vi "Actor Core.vi"(8 "error in":errorcluster, 11 "AverageCollector2D in":refnum<class "AverageCollector2D.lvclass">) -> (0 "error out":errorcluster, 3 "Actor out":refnum<class "Actor.lvclass">)   [LabVIEW 2014, in "AverageCollector2D.lvclass"]
doc: "(<B>Filename</B>: Actor Framework.lvlib:Actor.lvclass:Actor Core.vi)\n\nReceives messages to the actor, reacts to them, and initiates any error handling that may shut the actor down.\n\nDescendant classes may override this VI to append parallel tasks for the actor to complete while it handles messages. Overrides use the Call Parent Method node."
uses:
  AverageCollector2D.lvclass
  Framework/Collector/AbstractCollector2D/AbstractCollector2D.lvclass
  Framework/Interfaces/Viewable Actor/Viewable Actor.lvclass
  <vilib>/ActorFramework/Message Enqueuer/Message Priority.ctl
  <vilib>/ActorFramework/Message Enqueuer/Message Enqueuer.lvclass
  Framework/Collector/AbstractCollector/AbstractCollector Messages/Write Needed Number Msg/Write Needed Number Msg.lvclass
  Framework/Collector/AbstractCollector/AbstractCollector Messages/Reset Msg/Reset Msg.lvclass
  <vilib>/ActorFramework/Actor/Actor.lvclass
  Framework/Interfaces/Observable Actor/Observable Actor.lvclass
  Framework/Collector/AbstractCollector/AbstractCollector.lvclass
  Framework/Model/Data/Data2D/Data2D.lvclass
  Framework/Collector/AbstractCollector2D/Data2D Cluster.ctl
panel:
  out "Collected number":u32
  out "Stop":bool=TRUE
  in  "Needed number":u32=1
  in  "Reset":bool
  out "Intermediate result":dbl[][](graph)
  out "Data in":dbl[][](graph)
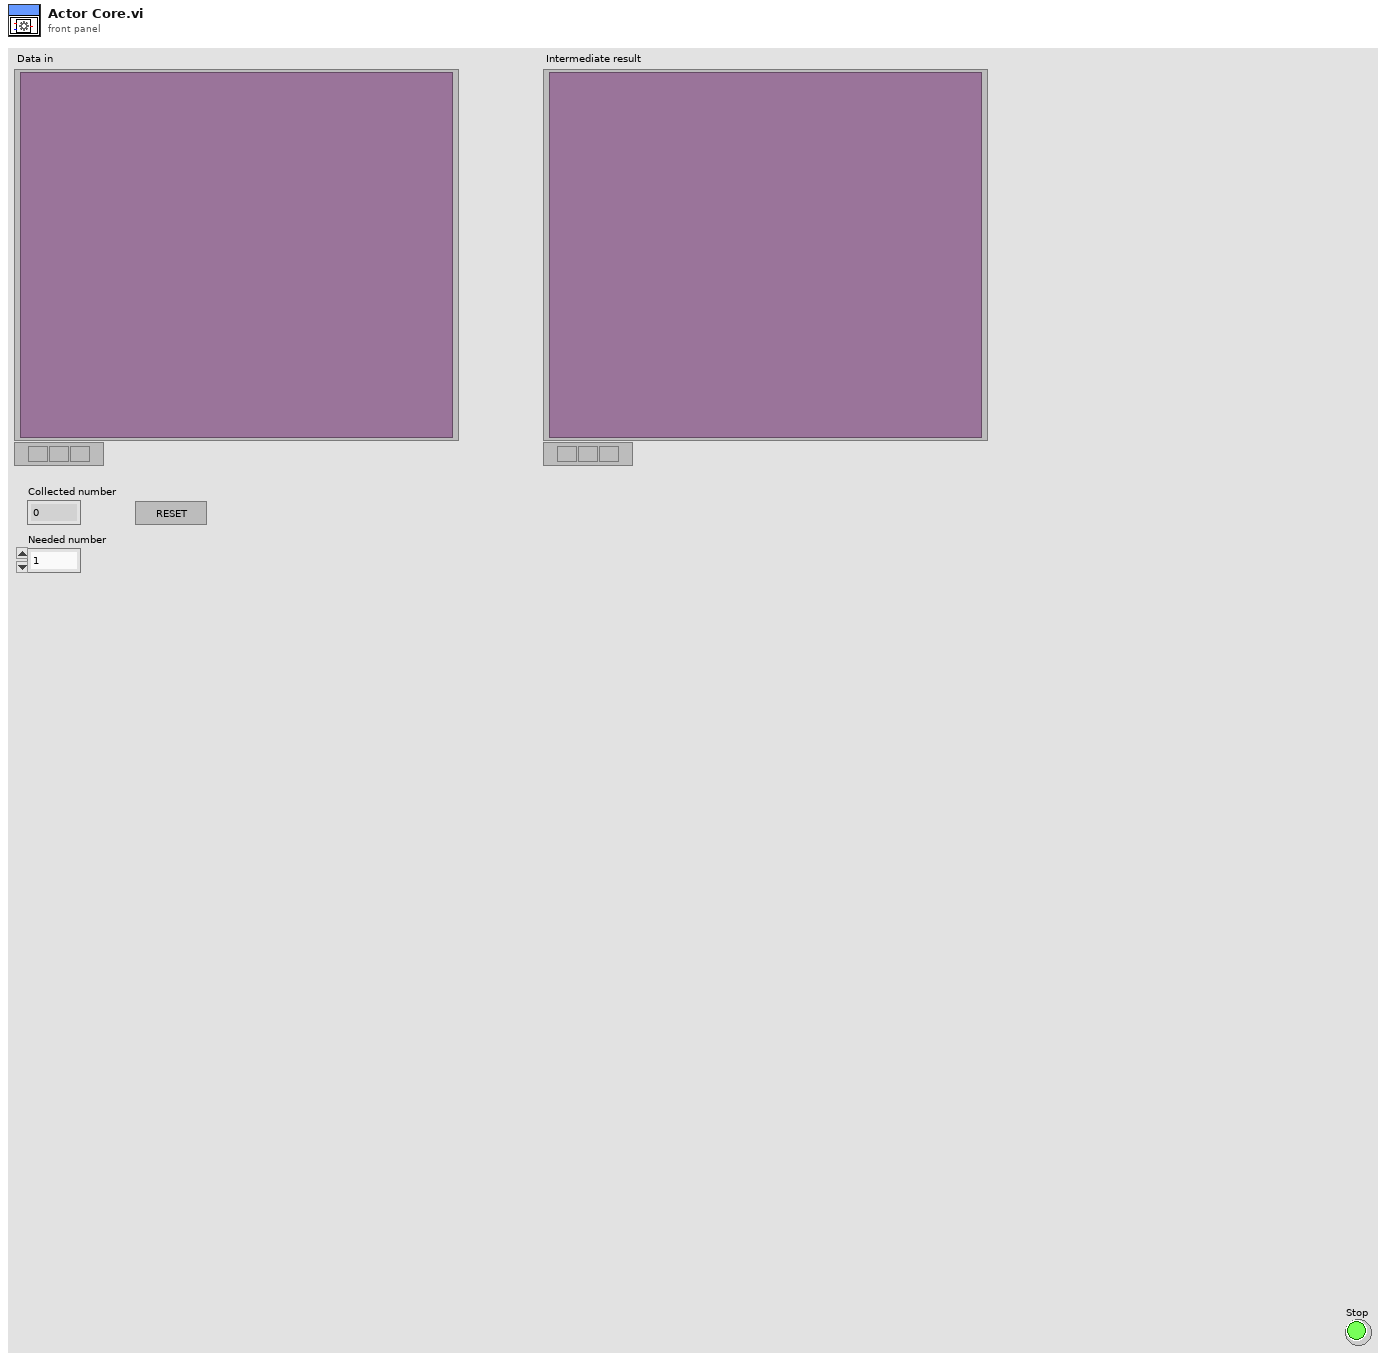
[diagram p1: front panel]
types:
  T1 = typedef "Observable Actor.lvlib/Observable Actor.lvclass/Observer.ctl" = refnum<queue>
  T2 = typedef "AbstractCollector2D.lvclass/Data2D Cluster.ctl" = cluster{"in":refnum<class "Data2D.lvclass">, "intermediate":refnum<class "Data2D.lvclass">}
  T3 = typedef "Actor Framework.lvlib/Message Enqueuer.lvclass/Message Priority.ctl" = enum16{"Low", "Normal", "High"}
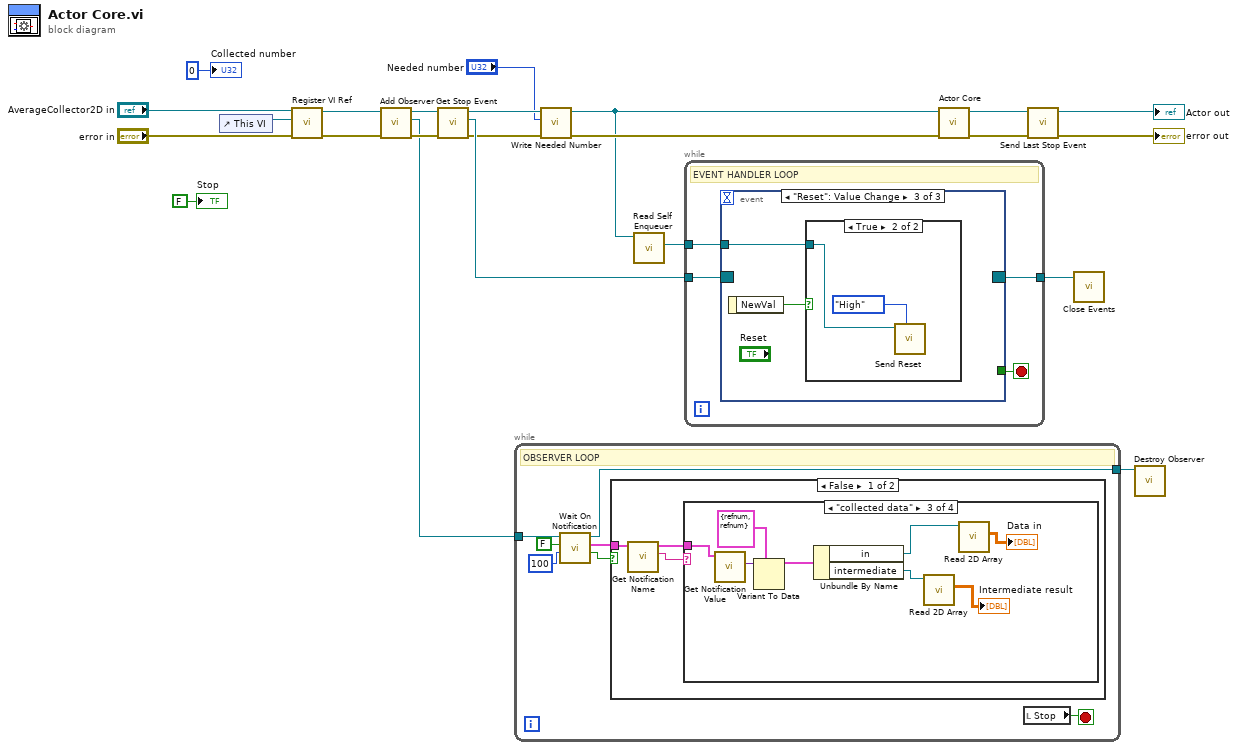
[diagram p0: block diagram]
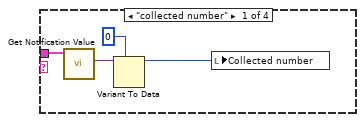
[diagram p2: hidden frame]
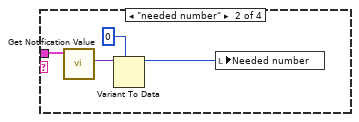
[diagram p3: hidden frame]
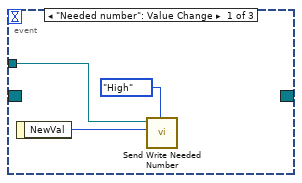
[diagram p6: hidden frame]
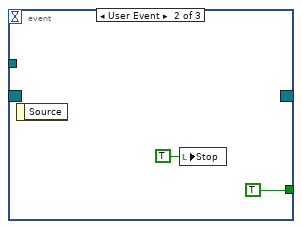
[diagram p7: hidden frame]
diagram:
  n1 = control-ref of="This VI"() -> (w23:refnum<vi>)
  n2 = call "Register VI Ref.vi"("error in (no error)"="error in", "VI ref"=w23, "Viewable Actor in"="AverageCollector2D in") -> ("error out"=w19:errorcluster, "Viewable Actor out"=w20:refnum<class "AverageCollector2D.lvclass">)  [unwired: 7 in]
  n3 = call-dynamic "Add Observer.vi"("error in (no error)"=w19, "Observable Actor in"=w20) -> ("error out"=w17:errorcluster, "new observer"=w10:T1, "Observable Actor out"=w18:refnum<class "AverageCollector2D.lvclass">)  [unwired: 7 in]
  n4 = call-dynamic "Get Stop Event.vi"("error in (no error)"=w17, "Observable Actor in"=w18) -> ("error out"=w7:errorcluster, "Events"=w16:refnum<event-registration>, "Observable Actor out"=w9:refnum<class "AverageCollector2D.lvclass">)  [unwired: 7 in]
  n5 = while {
    tunnel: w10 -> [w29]
    tunnel: [w24] -> w12
    stop <- w30 stop-if-true
    # "OBSERVER LOOP"
    n6 = call "Wait On Notification.vi"("timeout in ms (-1)"=100, "ignore previous (F)"=FALSE, "observer in"=w29) -> ("timed out?"=w25:bool, "notification"=w26:cluster{"value":variant, "name":string}, "observer out"=w24:T1)  [unwired: 5 in, 1 out]
    n7 = case shown="False" w25 {
      tunnel: w26 -> [w33 _]
      frame False {
        n8 = call "Get Notification Name.vi"("notification in"=w33) -> ("name"=w31:string, "notification out"=w32:cluster{"value":variant, "name":string})  [unwired: 9 in]
        n9 = case shown="\"collected data\"" w31 {
          tunnel: w32 -> [w37 w41 w47 _]
          frame "collected number" {
            n10 = call "Get Notification Value.vi"("notification in"=w37) -> ("data"=w36:variant)  [unwired: 7 in, 1 out]
            n11 = Variant To Data(type=u32 0, Variant=w36) -> (data=w34:u32)  [unwired: 1 in, 1 out]
            n12 = local write "Collected number"(w34) -> ()
          }
          frame "needed number" {
            n13 = call "Get Notification Value.vi"("notification in"=w41) -> ("data"=w40:variant)  [unwired: 7 in, 1 out]
            n14 = Variant To Data(type=u32 0, Variant=w40) -> (data=w38:u32)  [unwired: 1 in, 1 out]
            n15 = local write "Needed number"(w38) -> ()
          }
          frame "collected data" {
            n16 = call "Get Notification Value.vi"("notification in"=w47) -> ("data"=w49:variant)  [unwired: 7 in, 1 out]
            n17 = Variant To Data(type=T2 {"in"=refnum, "intermediate"=refnum} ("Cluster"), Variant=w49) -> (data=w48:T2)  [unwired: 1 in, 1 out]
            n18 = Unbundle By Name(w48) -> ("in"=w45:refnum<class "Data2D.lvclass">, "intermediate"=w46:refnum<class "Data2D.lvclass">)
            n19 = call "Read 2D Array.vi"("Data2D in"=w46) -> ("2D Array"=→"Intermediate result":dbl[][])  [unwired: 8 in, 2 out]
            n20 = call "Read 2D Array.vi"("Data2D in"=w45) -> ("2D Array"=→"Data in":dbl[][])  [unwired: 8 in, 2 out]
          }
          frame Default {
          }
        }
      }
      frame True {
      }
    }
    n21 = local read "Stop"() -> (w30:bool)
  }
  n22 = call "Write Needed Number.vi"("error in (no error)"=w7, "Needed Number"="Needed number", "AbstractCollector in"=w9) -> ("error out"=w6:errorcluster, "AbstractCollector out"=w5:refnum<class "AverageCollector2D.lvclass">)  [unwired: 7 in]
  n23 = call <vilib>:"Read Self Enqueuer.vi"("Actor"=w5) -> ("Self Enqueuer"=w22:refnum<class "Message Enqueuer.lvclass">)  [unwired: 10 in]
  n24 = while {
    tunnel: w16 -> [w53]
    tunnel: w22 -> [w52]
    tunnel: [w51] -> w13
    stop <- w50 stop-if-true
    # "EVENT HANDLER LOOP"
    n25 = event shown="[2] \"Reset\": Value Change" {
      selector: w53 -> [_ _ _]
      dyn-events: [_ _ _] -> w51
      timeout: _ -> [_ _ _]
      tunnel: w52 -> [w55 _ w59]
      tunnel: [_ TRUE _] -> w50
      event "Needed number": Value Change {
        n26 = event-data() -> ("NewVal"=w54:u32)  [unwired: 1 in]
        n27 = call "Send Write Needed Number.vi"("Message Priority (Normal)"=Message_Priority."High", "Needed Number"=w54, "Message Enqueuer"=w55) -> ()  [unwired: 7 in, 2 out]
      }
      event User Event {
        n28 = event-data() -> ()  [unwired: 1 in, 1 out]
        n29 = local write "Stop"(TRUE ("Stop")) -> ()
      }
      event "Reset": Value Change {
        n30 = event-data() -> ("NewVal"=w60:bool)  [unwired: 1 in]
        n31 = case shown="True" w60 {
          tunnel: w59 -> [_ w62]
          frame False {
          }
          frame True {
            n32 = call "Send Reset.vi"("Message Priority (Normal)"=Message_Priority."High", "Message Enqueuer"=w62) -> ()  [unwired: 8 in, 2 out]
          }
        }
      }
    }
  }
  n33 = call-parent "Actor Core.vi"("error in"=w6, "Actor in"=w5) -> ("error out"=w14:errorcluster, "Actor out"=w15:refnum<class "Actor.lvclass">)  [unwired: 8 in]
  n34 = call "Send Last Stop Event.vi"("error in (no error)"=w14, "Actor in"=w15) -> ("error out"=→"error out":errorcluster, "Actor  out"=→"Actor out":refnum<class "Actor.lvclass">)  [unwired: 8 in]
  n35 = call "Close Events.vi"("events"=w13) -> ()  [unwired: 11 in]
  n36 = call "Destroy Observer.vi"("observer in"=w12) -> ()  [unwired: 11 in]
  "Stop" <- FALSE ("Stop")
  "Collected number" <- u32 0 ("Collected number")
